vi "GetTestSetDef.vi"(6 "Legacy (f)?":bool, 8 "error in (no error)":errorcluster) -> (0 "error out":errorcluster, 2 "TestSetDef":T1={"General"={"ID"=0, "Model"="", "Dual Port?"=FALSE, "Options"="", "Options"={"E"=FALSE, "K"=FALSE, "H"=FALSE, "W"=FALSE, "F"=FALSE}, "Cal File"=path ""}, "Receiver"={"Fstart, MHz"=0.0, "Fstop MHz"=0.0, "Fstep MHz"=0.0, "IF, MHz"=0.0}, "RX Band"={"Fstart, MHz"=0.0, "Fstop MHz"=0.0}, "TX 1"={"Fstart, MHz"=0.0, "Fstop MHz"=0.0, "Pmax, dBm"=0.0, "Pstep, dB"=0.0}, "TX 2"={"Fstart, MHz"=0.0, "Fstop MHz"=0.0, "Pmax, dBm"=0.0, "Pstep, dB"=0.0}, "Low-side?"=TRUE})   [LabVIEW 2011]
uses:
  Test Set Definition.ctl
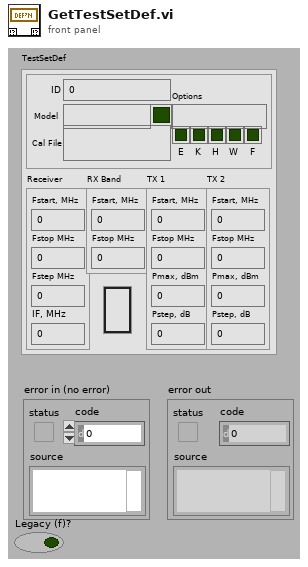
[diagram p1: front panel]
types:
  T1 = typedef "Test Set Definition.ctl" = cluster{"General":cluster{"ID":u32, "Model":string, "Dual Port?":bool, "Options":string, "Options":cluster{"E":bool, "K":bool, "H":bool, "W":bool, "F":bool}, "Cal File":path}, "Receiver":cluster{"Fstart, MHz":dbl, "Fstop MHz":dbl, "Fstep MHz":dbl, "IF, MHz":dbl}, "RX Band":cluster{"Fstart, MHz":dbl, "Fstop MHz":dbl}, "TX 1":cluster{"Fstart, MHz":dbl, "Fstop MHz":dbl, "Pmax, dBm":dbl, "Pstep, dB":dbl}, "TX 2":cluster{"Fstart, MHz":dbl, "Fstop MHz":dbl, "Pmax, dBm":dbl, "Pstep, dB":dbl}, "Low-side?":bool}
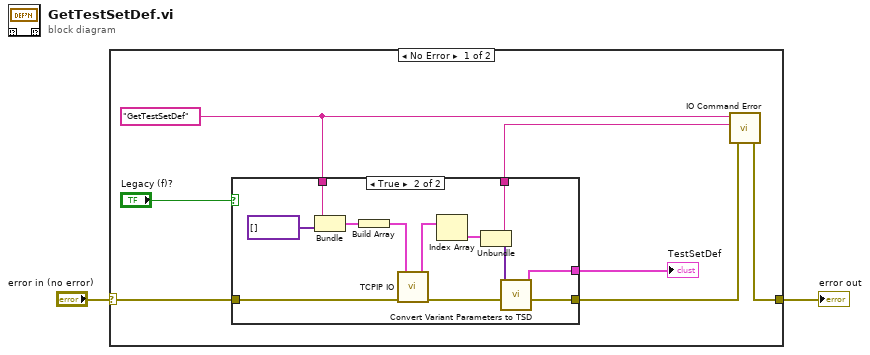
[diagram p0: block diagram]
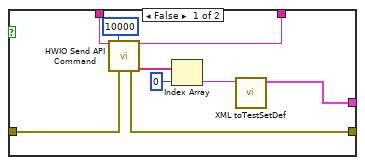
[diagram p2: hidden frame]
diagram:
  n1 = case shown="No Error" "error in (no error)" {
    selector: "error in (no error)" -> [w6 w31]
    tunnel: [w7 w31] -> w2
    frame No Error {
      w9 = "GetTestSetDef"
      n2 = case shown="True" "Legacy (f)?" {
        tunnel: w9 -> [w15 w29]
        tunnel: [w16 w28] -> w8
        tunnel: w6 -> [w18 w24]
        tunnel: [w17 w22] -> w5
        tunnel: [w10 w21] -> w4
        frame False {
          n3 = call "HWIO Send API Command.vi"("Action"=w15, "Timeout ms (5000)"=10000 ("PerCommand Timeout (ms)"), "error in (no error)"=w18) -> ("Action out"=w16:string, "error out"=w17:errorcluster, "String out"=w14:string[])  [unwired: 5 in, 5 out]
          n4 = Index Array(array=w14, index=0) -> (element=w11:string)
          n5 = call "XML toTestSetDef.vi"("TSD XML"=w11) -> ("Test Set Definition"=w10:T1)  [unwired: 10 in]
        }
        frame True {
          n6 = Bundle(w29, "appended array"=variant[] []) -> (w30:cluster{string, "appended array":variant[]})  [unwired: 1 out]
          n7 = Build Array(w30) -> (w25:cluster{string, "appended array":variant[]}[])
          n8 = call "TCPIP IO.vi"("error in (no error)"=w24, "Commands"=w25) -> ("error out"=w23:errorcluster, "Responses"=w27:cluster{string, variant[]}[])  [unwired: 1 in, 3 out]
          n9 = Index Array(array=w27) -> (element=w26:cluster{string, variant[]})  [unwired: 1 in]
          n10 = Unbundle(w26) -> (w28:string, w20:variant[])
          n11 = call "Convert Variant Parameters to TSD.vi"("error in"=w23, "Variant Parameter Array"=w20) -> ("error out"=w22:errorcluster, "TestSetDef"=w21:T1)  [unwired: 8 out]
        }
      }
      "TestSetDef" <- w4
      n12 = call "IO Command Error.vi"("error in (no error)"=w5, "Command Returned (\"\")"=w8, "Command Sent (\"\")"=w9) -> ("error out"=w7:errorcluster)  [unwired: 4 out]
    }
    frame Error {
    }
  }
  "error out" <- w2
